vi "JPL Lidar PID (SubVI).vi"(4 "Lidar Ref name":string, 5 "Distance Config":T2, 6 "PID Settings":T4, 7 "PID Limits":cluster{"Upper Limit":dbl, "Lower Limit":dbl}) -> (0 "Lidar Status":T3, 3 "output":dbl)   [LabVIEW 2014]
uses:
  <vilib>/Rock Robotics/WPI/Ultrasonic/WPI_SonarMB1010AnalogRefNum Registry Get.vi
  <vilib>/Rock Robotics/WPI/Ultrasonic/WPI_SonarMB1010AnalogGetRange.vi
  <vilib>/addons/control/pid/pid.llb/PID (DBL).vi
  <vilib>/addons/control/pid/NI_PID_pid.lvlib
panel:
  out "Sonar Status":T1
  in  "Sonar Ref name":string
  out "Distance Chart (Inches)":dbl(graph)
  out "PID Output Chart":dbl(graph)
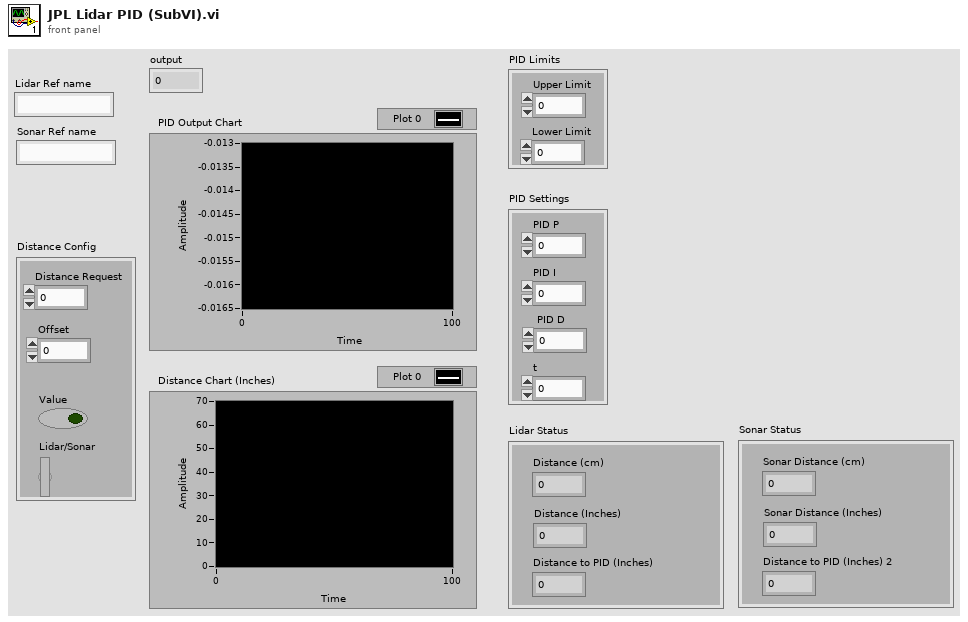
[diagram p1: front panel]
types:
  T1 = cluster{"Sonar Distance (cm)":dbl, "Sonar Distance (Inches)":dbl, "Distance to PID (Inches) 2":dbl}
  T2 = cluster{"Distance Request":dbl, "Offset":dbl, "Value":bool, "Lidar/Sonar":bool}
  T3 = cluster{"Distance (cm)":dbl, "Distance (Inches)":dbl, "Distance to PID (Inches)":dbl}
  T4 = cluster{"PID P":dbl, "PID I":dbl, " PID D":dbl, "t":dbl}
  T5 = typedef "WPI_I2CDevRef.ctl" = cluster{"DevStatus":errorcluster, "Controller":T6, "Device Address":u8, "Handle":i32, "I2C Bus":T7}
  T6 = typedef "FPGA_TypedefDigitalModule.ctl" = enum16{"Controller 1"}
  T7 = typedef "i2c_bus.ctl" = enum16{"I2C On-Board", "I2C MXP", "Invalid"}
  T8 = typedef "WPI_SonarMB1010AnalogDeviceRef.ctl" = cluster{"AIDeviceRef":T9, "Scaling factor (V/in)":dbl, "Average Bits":u8}
  T9 = typedef "WPI_AnalogChannelDevRef.ctl" = cluster{"DevStatus":errorcluster, "Controller":T10, "Analog Channel":T11}
  T10 = typedef "FPGA_TypedefAnalogModule.ctl" = enum16{"Controller 1"}
  T11 = typedef "FPGA_AIChannel.ctl" = enum8{"AI 0", "AI 1", "AI 2", "AI 3", "AI MXP 0", "AI MXP 1", "AI MXP 2", "AI MXP 3", "Invalid"}
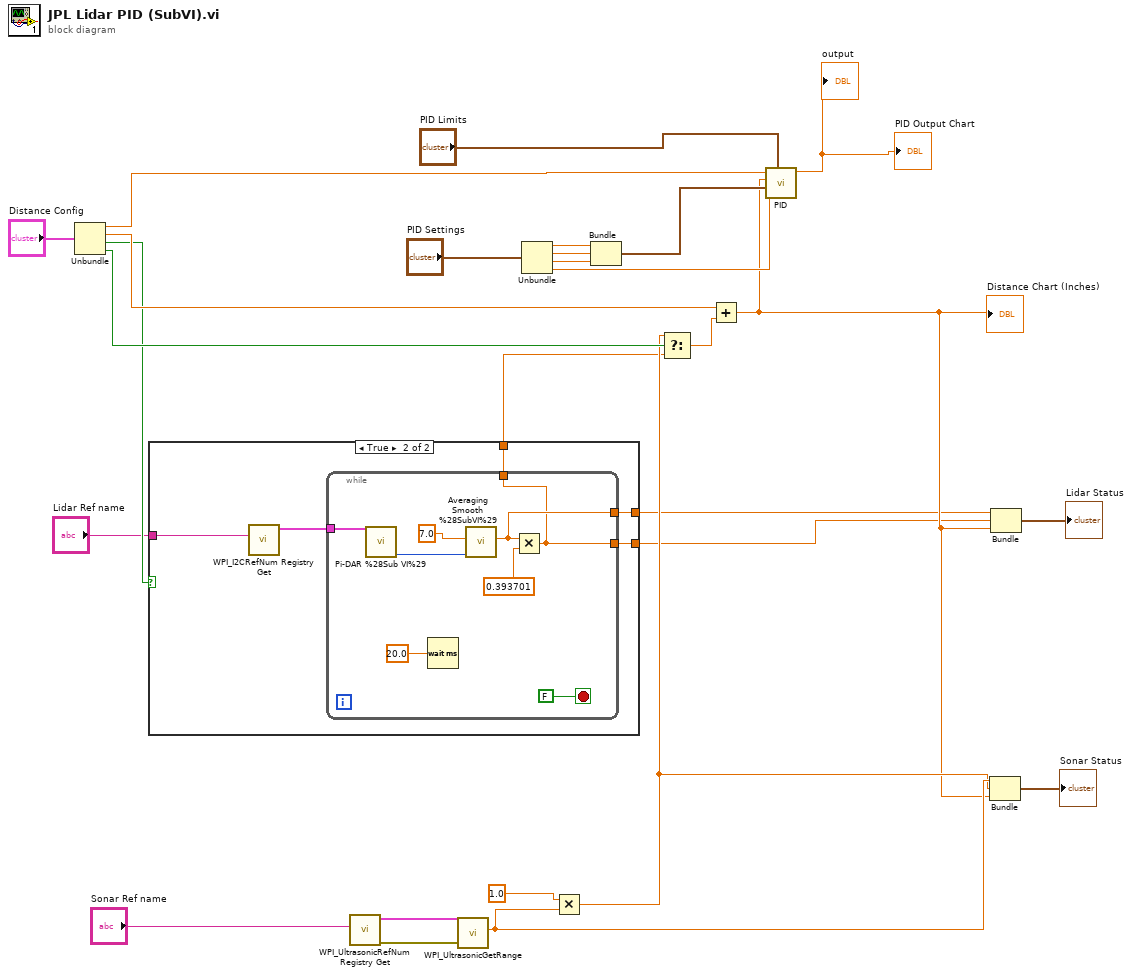
[diagram p0: block diagram]
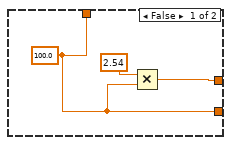
[diagram p2: hidden frame]
diagram:
  n1 = Unbundle("Distance Config") -> ("Distance Request"=w16:dbl, "Offset"=w17:dbl, "Value"=w8:bool, "Lidar/Sonar"=w15:bool)
  n2 = case shown="True" w8 {
    tunnel: [w29 w34] -> w7
    tunnel: [w30 w33] -> w3
    tunnel: [w29 w32] -> w2
    tunnel: "Lidar Ref name" -> [_ w31]
    frame False {
      w29 = 100.0
      n3 = Multiply(x=2.54, y=w29) -> (x*y=w30:dbl)
    }
    frame True {
      n4 = call <vilib>:"WPI_I2CRefNum Registry Get.vi"("refnum name"=w31) -> ("I2CDevRef"=w35:T5)  [unwired: 9 in, 1 out]
      n5 = while {
        tunnel: w35 -> [w39]
        tunnel: [w36] -> w34
        tunnel: [w37] -> w33
        tunnel: [w36] -> w32
        stop <- FALSE stop-if-true
        n6 = call "Pi-DAR %28Sub VI%29.vi"("I2CDevRef"=w39) -> ("Distance Output"=w43:i32)  [unwired: 10 in]
        n7 = Wait (ms)(milliseconds to wait=20.0) -> ()  [unwired: 1 out]
        n8 = call "Averaging Smooth %28SubVI%29.vi"("Input"=w43, "# of Samples to Average"=7.0) -> ("Output"=w37:dbl)  [unwired: 6 in, 1 out]
        n9 = Multiply(x=w37, y=0.393701) -> (x*y=w36:dbl)
      }
    }
  }
  n10 = call-poly <vilib>:"WPI_UltrasonicRefNum Registry Get.vi"("refnum name"="Sonar Ref name") -> ("error out"=w5:errorcluster, "SonarMB1010AnalogDevRef"=w6:T8)  [unwired: 9 in]
  n11 = call-poly <vilib>:"WPI_UltrasonicGetRange.vi"("error in"=w5, "SonarMB1010AnalogDevRef"=w6) -> ("Distance"=w11:dbl)  [unwired: 7 in, 2 out]
  n12 = Unbundle("PID Settings") -> ("PID P"=w24:dbl, "PID I"=w23:dbl, "PID D"=w22:dbl, "t"=w21:dbl)
  n13 = Multiply(x=1.0, y=w11) -> (x*y=w10:dbl)
  n14 = Bundle("PID P"=w24, "PID I"=w23, "PID D"=w22) -> (w20:cluster{"PID P":dbl, "PID I":dbl, " PID D":dbl})  [unwired: 1 in]
  n15 = Select(t=w10, s=w15, f=w7) -> (s? t:f=w14:dbl)
  n16 = Add(x=w17, y=w14) -> (x+y=w9:dbl)
  "Distance Chart (Inches)" <- w9
  n17 = call-poly <vilib>:"PID.vi"("output range"="PID Limits", "dt (s)"=w21, "PID gains"=w20, "process variable"=w9, "setpoint"=w16) -> ("output"=→"PID Output Chart" →"output":dbl)  [unwired: 5 in, 1 out]
  n18 = Bundle("Distance"=w11, w10, w9) -> (→"Sonar Status":cluster{"Distance":dbl, dbl, dbl})  [unwired: 1 in]
  n19 = Bundle("Output"=w3, w2, w9) -> (→"Lidar Status":cluster{"Output":dbl, dbl, dbl})  [unwired: 1 in]
